vi "HFRR ADV v017 new software.vi"() -> ()   [LabVIEW 2025] (continued)
  # "µm"
  # "Calibration Centre\nSelect a calibration procedure to begin. Each procedure guides you through all required steps."
  # "Apply known deadweight loads to validate \nthe friction force measurement chain \nand compute the calibration factor for the f\norce transducer."
  # "Step-by-step guided displacement calibration \nacross 6 positions from 0.1 mm to 1.2 mm. Tear \nfirst, then measure each position one by one."
  # "Two-set calibration: one point at 0 °C \nice-point) and one at 60 °C (high-point) \nusing a  reference Calibrator."
  # "Step 1 — Pre-calibration Setup"
  # "Prepare the displacement calibration reference gauge. Ensure the LVDT sensor is connected and the carriage slides freely. You will be guided through 6 positions from 0.2 mm to 1.2 mm, one at a time"
  # "Step 7 — Tare ( ZERO REFERENCE )"
  # "Before measuring, the sensor must be zeroed. Move the carriage to the mechanical zero stop — no displacement applied. Once in position, tap Tare & Begin to zero the reference."
  # "Step 8 — POSITION MEASUREMENT"
  # "Measurement Checklist"
  # "Position the carriage at exactly this \nvalue using your reference gauge, then tap Confirm &\n Next."
  # "All 6 positions recorded!\n\nTap Confirm & Next  to review the calibration summary."
  # "Step 9 — CALIBRATION RESULT"
  # "Stroke Calibration Complete\nAll 6 positions (0.2 mm – 1.2 mm)"
  # "Calibrates the sample/bath temperature sensor. \nUsed for test specimen and lubricant temperature measurement."
  # "Calibrates the ambient air temperature sensor. \nUsed for environmental chamber monitoring."
  # "Set B\n60 °C\nHigh-point calibration"
  # "Set A\n0 °C\nIce-point calibration"
  # "Set B\n60 °C\nHigh-point calibration"
  # "Set A\n0 °C\nIce-point calibration"
  # "Select Temperature Sensor"
  # "Choose which temperature sensor you are calibrating. Both use the same two-\npoint procedure: 0 °C (ice-point) and 60 °C (high-point)."
  # "Step 1 — Reference Instrument Setup"
  # "Connect a calibrated reference to the DUT port. This calibration performs two sets: one at 0 °C and one at 60 °C."
  # "Set A\n0 °C\nIce-point calibration"
  # "Set B\n60 °C\nHigh-point calibration"
  # "Allow the temperature bath to stabilise for at least 2 minutes at each set-point before recording the reading."
  # "Step 2 — Set A:  0 °C Calibration"
  # "Connect the  0 °C reference connector. Wait for the temperature to stabilise. Once stable, and click Record Point."
  # "Step 3 — Set A:  60 °C Calibration"
  # "Connect the  60 °C reference connector. Wait for the temperature to stabilise. Once stable, and click Record Point."
  # "Step 1 — Reference Instrument Setup"
  # "Connect a calibrated reference to the DUT port. This calibration performs two sets: one at 0 °C and one at 60 °C."
  # "Set A\n0 °C\nIce-point calibration"
  # "Set B\n60 °C\nHigh-point calibration"
  # "Allow the temperature bath to stabilise for at least 2 minutes at each set-point before recording the reading."
  # "Step 2 — Set A:  0 °C Calibration"
  # "Connect the  0 °C reference connector. Wait for the temperature to stabilise. Once stable, and click Record Point."
  # "Step 3 — Set A:  60 °C Calibration"
  # "Connect the  60 °C reference connector. Wait for the temperature to stabilise. Once stable, and click Record Point."
  # "System Control Commands\nS;1 - Starts the full automation cycle (Runs Priming-humidify till 70RH sequence first, then switches to Maintenance).\nS;0 - Stops the system immediately and enters Standby mode (Safe State: All actuators OFF).\nM;1 - Skips the priming sequence and jumps directly to Maintenance mode (PID control).\nR;1 - Resets the logic state machine and clears all errors, returning to Standby.\nService Mode (Manual Control)\nX;1 - Enters Manual Service Mode. This disables all automatic logic, sensor safety checks, and timers.\nX;0 - Exits Manual Service Mode and returns to Standby (Safe State).\nActuator Commands (Only work after sending X;1)\nP;[0-255] - Sets the Pump PWM. Note that this is Active Low (0 = Max Flow, 255 = Pump OFF).\nF;I;[0-255] - Sets the Intake Fan speed (0 = OFF, 255 = Max Speed).\nF;O;[0-255] - Sets the Exhaust Fan speed (0 = OFF, 255 = Max Speed).\nD;1 - Turns the Dehumidifier Relay ON.\nD;0 - Turns the Dehumidifier Relay OFF."
  # "%RH"
  # "ISO : WS1.4"
  # "Start test and end test log--- done\nDisable heater ON and Humidity ON during the test --- done\ntemprature and ---done\nhumidity reach log\nauto start run true logic and log\nmanual start log once"
  # "Reference Fluid Information"
  # "Note:\nMake sure to place all images in the folder \"C:\\WinDucom\\im\" before clicking on \"Import Image.\""
  # "NOTE:\nPlace all the images in the path \"C:\\WinDucom\\im\" before clicking on Import Image"
  # "Wear Scar Measurements"
  # "Reference Fluid Information"
  # "Graph :"
types:
  T1 = enum32{"Home", "Dashboard", "Imaging", "Report", "Analysis", "About", "Test Setup", "Advance", "Calibration"}
  T2 = enum32{"HOME", "Test Setup", "Acquire", "Adv Scar", "Adv Scar Report", "Compare Files", "Calibration", "About", "Advance", "Mooha"}
  T3 = enum16{"ASTM D6079", "ISO 12156", "CEC F-096-A-06", "Custom"}
  T4 = enum32{"Dashboard 1", "Dashboard 2", "Dashboard 3"}
  T5 = enum32{"COF", "Friction", "ECR", "Temperature", "Humidity", "Stroke"}
  T6 = enum32{"Coefficient Of Friction", "Air Temperature", "Humidity", "Stroke", "Sample Temperature", "Electrical Contact Resistance", "Frequency", "Air Temp vs Rh"}
  T7 = enum32{"Main", "Stroke", "Friction", "Temperature"}
  T8 = enum32{"Stroke Calibration", "Friction Force Calibration", "Temperature Calibration"}
  T9 = enum32{"Step 1", "Step 2", "Step 3", "Step 4", "Step 5", "Step 6", "Step 7", "Step 8", "Step 9"}
  T10 = enum32{"Test Progress", "Stroke Points Completed"}
  T11 = enum32{"Main", "Step 1", "Step 2", "Step 3", "Air Step 1", "Air Step 2", "Air Step 3"}
  T12 = enum32{"Gains", "Configuration Parameters", "Temperature Calibration"}
  T13 = enum32{"Stroke Data", "Temperature Calibration", "Friction Force Raw Data"}
  T14 = enum32{"Temp Variables", "Camera", "WO 2465 (1)", "WO 2465 (2)", "WO 2465 (3)"}
  T15 = typedef "Auto Start enum.ctl" = enum16{"Init", "Humidity & Temperature On", "Reach point", "Maintain Stage", "Start Stage", "close", "Exit"}
  T16 = typedef "imagedata.ctl" = cluster{"image type":i32, "image depth":i32, "image":u8[], "mask":u8[], "colors":u32[], "Rectangle":cluster{"left":i16, "top":i16, "right":i16, "bottom":i16}}
  T17 = enum32{"HOME", "Test Setup", "Acquire", "Compare Files", "Print Report", "About", "Advance", "Mooha"}
  T18 = cluster{"Read Heave and Surge":string, "Bytes at Heave Port":dbl, "Heave and Surge COM Port:":refnum<visa-resource-name>, "Com Port 2":refnum<visa-resource-name>, "Residual Due":string, "Heave COM Status 2":bool, "Heave COM Status":bool, "Port 2":bool, "Sway PPR":dbl, "Surge PPR":dbl, "Heave PPR":dbl, "Sway Pitch":dbl, "Surge Pitch":dbl, "Heave Pitch":dbl, "Sway Pulses/mm":dbl, "Surge Pulses/mm":dbl, "Heave Pulses/mm":dbl, "inner loop":dbl, "Read Heave and Surge 2":string, "String 36":string, "Write S":bool, "WriteCC1":string[], "Heave COM Loop":i32, "LastCom":string, "EXIT":bool, "Error Heave":errorcluster}
  T19 = enum8{"Enabled", "Disabled", "Disabled and Grayed Out"}
  T20 = enum32{"HOME", "Test Setup", "Acquire", "Adv Scar", "Adv Scar Report", "Compare Files", "About", "Advance", "Mooha"}
  T21 = enum16{"Always On", "Always Off", "Off While Running"}
  T22 = typedef "POST ANALYSIS ENUM.ctl" = enum16{"OPEN EXE", "INIT", "OPEN FILE", "FIT", "DRAW REC", "DRAW LINE", "PAN", "ZOOM IN", "ZOOM OUT", "SET ZOOM", "CLEAR ROI", "GET MEASUREMENTS", "RESIZE MODE", "STREAM START", "STREAM STOP", "SHOW UI", "MINIMIZE UI", "HIDE UI", "CKISE APP", "CLOSE CONNECTION", "SAVE IMAGE", "SET ROI COLOR", "READ", "TCP CHECK", "CLOSE"}
  T23 = typedef "CAMERA LIVE FEED ENUM.ctl" = enum16{"OPEN EXE", "INIT", "READ", "CAMERA CONNECT", "CAMERA START", "CAMERA STOP", "CAMERA GRAY", "CAMERA RGB", "CAMERA MINIMIZE", "CAMERA CLOSE", "CAMERA MODE LIST", "CAMERA MODE SET", "CAMERA RESTORE", "CAMERA SAVE", "CLOSE"}
  T24 = enum32{"Home", "Dashboard", "Imaging", "Report", "Analysis", "About", "Test Setup", "Advance"}
  T25 = cluster{"File Name":string, "Test Method":string, "Operator":string, "Fuel Description":string, "Date and time":string}
  T26 = enum32{"Home", "Dashboard", "Imaging", "Report", "Analysis", "About", "Test Setup"}
  T27 = enum32{"HOME", "Test Setup", "Acquire", "Compare Files", "About", "Advance", "Mooha"}
  T28 = enum16{"deny read/write", "deny write-only", "deny none"}
  T29 = typedef "NI_ReportGenerationCore.lvlib/HTML Report Image Alignment.ctl" = enum16{"(default)", "LEFT", "RIGHT", "TOP", "TEXTTOP", "MIDDLE", "ABSMIDDLE", "BASELINE", "BOTTOM", "ABSBOTTOM"}
  T30 = enum16{"open", "replace", "create", "open or create", "replace or create", "replace or create with confirmation"}
  T31 = enum16{"INIT", "READ", "MANUAL WRITE", "WRITE", "CLOSE", "ERROR INIT"}
  T32 = enum16{"open", "open or create", "create or replace", "create", "open (read only)"}
  T33 = cluster{"Mode":enum16{"RTU", "ASCII"}, "Slave Address":u8}
diagram:
  w11 = FALSE ("Visible")
  w12 = T19."Enabled" ("Disabled")
  w15 = FALSE ("Visible")
  w14 = FALSE ("Humidity Off Command")
  w32 = "" ("USER ID")
  (unwired) T20."HOME" ("Main Tab")
  # "[CH1]    - FF\n[CH2]   - TEMPERATURE\n[CH3]    - Humidity\n[CH4]    - AIR TEMP\n[CH5]\\- Visa Uno\n[CH6] \\- Visa Due\n[CH7]  \\- file path\n[CH8]   - Displacement Gain\n[CHA]   - Stroke Gain\n[CHB]   - Stroke PID Gain\n[CHC]   -Language Selection\n[CHD]   -Power +\n[CHE]   -Power_\n[CHF]   -Heater\n[CHG]   -Humidity Wet\n[CHH]   -Humidity Dry\n[CHI]   -Integral Time \n[CHIJ   -Air intercept\n[CHI]   -Temp Intercept"
  n1 = flat-sequence {
    tunnel: [w81] -> w24
    tunnel: w24 -> [w95]
    tunnel: [w94] -> w23
    tunnel: ["ao0"] -> w26
    tunnel: w23 -> [_]
    tunnel: w26 -> [w159]
    tunnel: [w159] -> w25
    tunnel: w25 -> [w205]
    tunnel: [w203] -> w36
    tunnel: [w205] -> w35
    tunnel: w36 -> [w255]
    tunnel: w35 -> [w212]
    tunnel: [w255] -> w22
    tunnel: [w218] -> w21
    tunnel: [w206] -> w20
    tunnel: [w261] -> _
    tunnel: [w260] -> _
    tunnel: [w262] -> w58
    tunnel: w22 -> [w262]
    tunnel: w21 -> [w260]
    tunnel: w20 -> [w261]
    frame #0 {
      n2 = disable-structure shown="Disabled" {
        frame Disabled {
          n3 = control-ref of="This VI"() -> (w69:refnum<vi>)
          n4 = property class="VI"(reference=w69) -> (reference out=w60:refnum<vi>, error out=w64:errorcluster, "Panel"=w68:refnum<vi>)  [unwired: 1 in]
          n5 = property class="Pnl"(reference=w68, error in=w64) -> (reference out=w62:refnum<vi>, error out=w65:errorcluster, "Panes[]"=w67:refnum<vi>[])
          n6 = for {
            tunnel: w67 -> [w75] mode=indexing
            tunnel: T21."Always Off" ("Horizontal Scrollbar Visibility") -> [w74]
            tunnel: w65 -> [w71]
            tunnel: [w70] -> w63
            n7 = property class="Pane"(reference=w75, error in=w71, "HorizScrollbarVisibility"=w74) -> (reference out=w72:refnum<vi>, error out=w73:errorcluster)
            n8 = Close Reference(reference=w72, error in (no error)=w73) -> (error out=w70:errorcluster)
          }
          n9 = Close Reference(reference=w62, error in (no error)=w63) -> (error out=w61:errorcluster)
          n10 = Close Reference(reference=w60, error in (no error)=w61) -> (error out=→"error out 8":errorcluster)
        }
        frame Enabled {
        }
      }
    }
    frame #1 {
      n11 = call "CLOSE CONNECTION.vi"("error in (no error)"="error in (no error) 2") -> ("error out"=w79:errorcluster)  [unwired: 10 in]
      n12 = call <vilib>:"Clear Errors.vi"("error in (no error)"=w79) -> ("error out"=w78:errorcluster)  [unwired: 5 in, 1 out]
      n13 = disable-structure shown="Enabled" {
        disable-tunnel: w78 -> [w85 _]
        disable-tunnel: [w84 _] -> w81
        frame Enabled {
          n14 = call <userlib>:"Fit VI window to Largest Dec.vi"("error in (no error)"=w85, "border spacing (2 px)"=1) -> ("error out"=w88:errorcluster, "dup VI Ref"=w92:refnum<vi>)  [unwired: 4 in]
          n15 = invoke on="Invoke Node" class="VI" method="FP.Run-Time Position.Maximized"(reference=w92, error in=w88) -> (error out=w89:errorcluster)  [unwired: 2 in, 3 out]
          n16 = call <vilib>:"Clear Errors.vi"("error in (no error)"=w89) -> ("error out"=w91:errorcluster)  [unwired: 5 in, 1 out]
          n17 = control-ref of="This VI"() -> (w83:refnum<vi>)
          n18 = invoke on="Invoke Node" class="VI" method="Default Vals.Reinit All"(reference=w83, error in=w91) -> (reference out=w87:refnum<vi>, error out=w86:errorcluster)  [unwired: 1 in, 1 out]
          n19 = Close Reference(reference=w87, error in (no error)=w86) -> (error out=w84:errorcluster)
        }
        frame Disabled {
        }
      }
      n20 = local write "sign in temp"(FALSE ("sign in temp")) -> ()
      n21 = property on="Sign In" class="Bool (strict)"("DisabledEnum"=T19."Disabled" ("Disabled")) -> ()  [unwired: 2 in, 2 out]
      n22 = property on="Auto Scar Check" class="Clust (strict)"("Visible"=TRUE) -> ()  [unwired: 2 in, 2 out]
    }
    frame #2 {
      n23 = call "dialog box.vi"("Status"="Before starting the test, verify that the microscope cable is connected.", "error in"=w95) -> ("error out"=w94:errorcluster)  [unwired: 8 in]
    }
    frame #3 {
      (unwired) TRUE ("Re-Initialise")
      w101 = FALSE ("Upld AR 2")
      # "kkkkk"
      # "C:\\Windows\\wndcm_pw_stdED hfrr.txt"
      # "C:\\LAB-IQ NXT"
      # "C:\\LAB-IQ NXT\\wndcm_pw_stdED hfrr.txt"
      # "password file"
      n24 = Current VI's Path() -> (path=w114:path)
      n25 = Strip Path(path=w114) -> (stripped path=w107:path)  [unwired: 1 out]
      n26 = Path To String(path=w107) -> (string=w109:string)
      n27 = local write "conststatus"(0.0 ("rpm value : 2")) -> ()
      n28 = local write "Upld AR 2"(TRUE ("Upld AR 2")) -> ()
      n29 = local write "Lan flag"(0.0 ("Lan flag")) -> ()
      n30 = local write "COUNT"(0 ("COUNT")) -> ()
      n31 = local write "FLAG 2"(0.0 ("FLAG 2")) -> ()
      n32 = local write "Com flag"(u32 0 ("Com flag")) -> ()
      n33 = local write "refresh flag"(FALSE ("refresh flag")) -> ()
      n34 = local write "Json St Flg"(w101) -> ()
      n35 = Search/Split String(string=w109, search string/char (-)=".exe") -> (match + rest of string=w111:string)  [unwired: 1 in, 2 out]
      n36 = Match True/False String(2:".vi" ("false string"), 3:".exe" ("true string"), 4:w111) -> (0:w108:bool)  [unwired: 1 out]
      n37 = local write "Json End Flg"(w101) -> ()
      n38 = case shown="True" w108 {
        tunnel: w107 -> [w130 w132]
        tunnel: [w130 w131] -> w105
        frame False {
        }
        frame True {
          n39 = Strip Path(path=w132) -> (stripped path=w131:path)  [unwired: 1 out]
        }
      }
      n40 = Path To String(path=w105) -> (string=→"Gain path":string)
      n41 = local write "Main Tab Display"(T4."Dashboard 1" ("Main Tab Display")) -> ()
      n42 = local write "main tab sub"(enum32{"Page 1", "Page 2"}."Page 1" ("main tab sub")) -> ()
      n43 = local write "Main Tab"(T2."HOME" ("Main Tab")) -> ()
      n44 = local write "EVENT LOG"("") -> ()
      n45 = List Folder(path=path "C:/LAB-IQ" ("directory path"), pattern="*.txt") -> (filenames=w120:string[])  [unwired: 2 in, 3 out]
      n46 = Search 1D Array(1D array=w120, element="wndcm_pw_stdED hfrr.txt") -> (index of element=w123:i32)  [unwired: 1 in]
      n47 = Equal?(x=w123, y=-1) -> (x = y?=w118:bool)
      n48 = case shown="True" w118 {
        frame False {
        }
        frame True {
          n49 = String To Byte Array(string="123\n") -> (unsigned byte array=w137:u8[])
          n50 = Array Size(array=w137) -> (size(s)=w136:i32)
          n51 = for {
            N: w136 -> [_]
            tunnel: w137 -> [w150]
            tunnel: [w147] -> w139 mode=indexing
            tunnel: w136 -> [w142]
            i -> [w140]
            n52 = Decrement(x=w142) -> (x-1=w143:i32)
            n53 = Equal?(x=w140, y=w143) -> (x = y?=w144:bool)
            n54 = Index Array(array=w150, index=w140) -> (element=w149:u8)
            n55 = Number To Decimal String(number=w149) -> (decimal integer string=w148:string)  [unwired: 1 in]
            n56 = Select(t="", s=w144, f="\r") -> (s? t:f=w141:string)
            n57 = Concatenate Strings(w148, w141) -> (w147:string)
          }
          n58 = local read "file path"() -> (w133:path)
          n59 = Concatenate Strings(w139) -> (w135:string)
          n60 = call <vilib>:"Write Characters To File.vi"("append to file? (new file:F)"=FALSE, "character string"=w135, "file path (dialog if empty)"=w133) -> ()  [unwired: 2 in, 1 out]
        }
      }
      n61 = local write "clk"(0.0 ("clk")) -> ()
      n62 = local write "Flag"(0.0 ("Flag")) -> ()
      "file path" <- path "C:/LAB-IQ/wndcm_pw_stdED hfrr.txt" ("file path")
      "FF buffer" <- dbl[] [] ("FF buffer")
    }
    frame #4 {
      # "C:\\WinDucom\\calibrate WO 2391.dcf"
      n63 = String To Path(string="C:\\LAB-IQ\\calibrate WO 2465.dcf") -> (path=w158:path)
      n64 = Open/Create/Replace File "Open File"(file path (use dialog)=w158) -> (refnum out=w157:refnum<file>)  [unwired: 5 in, 2 out]
      n65 = for {
        N: 24 -> [_]
        tunnel: w157 -> [w178]
        i -> [w172]
        (unwired) TRUE ("line mode (F)")
        n66 = Read from Text File "Read File"(file (use dialog)=w178) -> (text=w177:string)  [unwired: 3 in, 3 out]
        n67 = Match Pattern(string=w177, regular expression="]") -> (after substring=w175:string)  [unwired: 1 in, 3 out]
        n68 = String Subset(string=w177, offset (0)=5, length (rest)=10 ("length (rest)")) -> (substring=w170:string)
        n69 = Fract/Exp String To Number(string=w170) -> (number=w171:dbl)  [unwired: 3 in, 1 out]
        n70 = Match Pattern(string=w175, regular expression="-") -> (before substring=w173:string)  [unwired: 1 in, 3 out]
        n71 = case shown="19" w172 {
          tunnel: w171 -> [w181 w182 w183 w184 _ _ _ w189 w190 _ w191 w192 w193 w194 w195 w196 _ w197 w198 _ _ _ _ _ _]
          tunnel: w173 -> [_ _ _ _ w185 w186 w187 _ _ _ _ _ _ _ _ _ _ _ _ w199 w200 _ w201 w202 _]
          frame 0 {
            n72 = local write "FRIC. FORCE :"(w181) -> ()
          }
          frame 1 {
            n73 = local write "TEMPERATURE :"(w182) -> ()
          }
          frame 2 {
            n74 = local write "HUMIDITY:"(w183) -> ()
          }
          frame 3 {
            n75 = local write "AIR TEMPERATURE :"(w184) -> ()
          }
          frame 4 {
            n76 = local write "Com Port 1"(w185) -> ()
          }
          frame 5 {
            n77 = local write "Com Port 2"(w186) -> ()
            n78 = local write "visa due"(w186) -> ()
          }
          frame 6 {
            n79 = String To Path(string=w187) -> (path=w188:path)
            n80 = local write "File Path"(w188) -> ()
          }
          frame 7 {
            n81 = local write "DISPLACEMENT :"(w189) -> ()
          }
          frame 8 {
            n82 = local write "STROKE GAIN :"(w190) -> ()
          }
          frame 9 {
          }
          frame 10 {
            n83 = local write "Language Selection"(w191) -> ()
          }
          frame 11 {
            n84 = local write "CH-POWER +"(w192) -> ()
          }
          frame 12 {
            n85 = local write "CH-POWER -"(w193) -> ()
          }
          frame 13 {
            n86 = local write "CH-HEATER"(w194) -> ()
          }
          frame 14 {
            n87 = local write "CH-HUMIDITY WET"(w195) -> ()
          }
          frame 15 {
            n88 = local write "CH-HUMIDITY DRY"(w196) -> ()
          }
          frame 16 {
          }
          frame 17 {
            n89 = local write "AIR TEMP INTERCEPT:"(w197) -> ()
          }
          frame 18 {
            n90 = local write "TEMP INTERCEPT:"(w198) -> ()
          }
          frame 21 {
            n91 = local write "S.NO"(w199) -> ()
          }
          frame 22 {
            n92 = local write "Com Port 3"(w200) -> ()
          }
          frame 23 {
          }
          frame 19 {
            n93 = local write "C3 :"(w201) -> ()
          }
          frame 20 {
            n94 = local write "Camera Port :"(w202) -> ()
          }
          frame 24, Default {
          }
        }
      }
      n95 = String To Path(string="C:\\LAB-IQ\\Image Calibrate v01.dcf") -> (path=w154:path)
      n96 = Open/Create/Replace File ("Open File")(file path (use dialog)=w154) -> (refnum out=w153:refnum<file>)  [unwired: 5 in, 2 out]
      n97 = for {
        N: 4 -> [_]
        tunnel: w153 -> [w165]
        i -> [w161]
        n98 = Read from Text File ("Read File")(file (use dialog)=w165) -> (text=w166:string)  [unwired: 3 in, 3 out]
        n99 = String Subset(string=w166, offset (0)=6, length (rest)=10 ("length (rest)")) -> (substring=w162:string)
        n100 = Fract/Exp String To Number(string=w162) -> (number=w160:dbl)  [unwired: 3 in, 1 out]
        n101 = case shown="3" w161 {
          tunnel: w160 -> [w167 w168 _ w169 _]
          frame 0 {
            n102 = local write "5x Gain"(w167) -> ()
          }
          frame 1 {
            n103 = local write "10x Gain"(w168) -> ()
          }
          frame 2 {
          }
          frame 3 {
            n104 = local write "100x gain"(w169) -> ()
          }
          frame 4, Default {
          }
        }
      }
    }
    frame #5 {
      n105 = Wait (ms)(milliseconds to wait=u32 1000) -> (millisecond timer value=w203:u32)
    }
    frame #6 {
      w221 = u32 2000 ("milliseconds to wait")
      w248 = u32 2000 ("milliseconds to wait")
      n106 = call "CAMERA LIVE FEED FGV.vi"("Enum - Menu"=CAMERA_LIVE_FEED_ENUM."OPEN EXE", "error in (no error)"=w212) -> ("error out"=w254:errorcluster)  [unwired: 8 in, 1 out]
      n107 = call "Stall Data Flow.vim"("value in"=w254, "milliseconds to wait"=w248) -> ("value out"=w252:errorcluster)  [unwired: 1 out]
      n108 = call "CAMERA LIVE FEED FGV.vi"("Enum - Menu"=CAMERA_LIVE_FEED_ENUM."INIT", "error in (no error)"=w252) -> ("error out"=w250:errorcluster)  [unwired: 8 in, 1 out]
      n109 = call "IMAGE ANALYSIS.vi"("Enum"=POST_ANALYSIS_ENUM."OPEN EXE", "error in"=w212) -> ("error out"=w209:errorcluster)  [unwired: 8 in, 1 out]
      n110 = case shown="Error .." w250 {
        selector: w250 -> [w256 _]
        tunnel: [w256 _] -> w249
        frame No Error {
        }
        frame Error {
          n111 = One Button Dialog(message="Camera initialization error.\nPlease Restart the software") -> ()  [unwired: 1 in, 1 out]
        }
      }
      n112 = call "Stall Data Flow.vim"("value in"=w209, "milliseconds to wait"=u32 8000) -> ("value out"=w208:errorcluster)  [unwired: 1 out]
      n113 = property on="Camera Port :" class="CmbBox"() -> ("Strings[]"=w246:string[], "Value"=w247:string)  [unwired: 2 in, 2 out]
      n114 = call "IMAGE ANALYSIS.vi"("Enum"=POST_ANALYSIS_ENUM."INIT", "error in"=w208) -> ("error out"=w206:errorcluster)  [unwired: 8 in, 1 out]
      n115 = Search 1D Array(1D array=w246, element=w247) -> (index of element=w245:i32)  [unwired: 1 in]
      n116 = Type Cast(type=30, x=w245) -> (*(type *) &x=w243:i32)
      n117 = call "Stall Data Flow.vim"("value in"=w249, "milliseconds to wait"=w248) -> ("value out"=w225:errorcluster)  [unwired: 1 out]
      n118 = Add(x=w243, y=48) -> (x+y=w224:i32)
      n119 = call "CAMERA LIVE FEED FGV.vi"("Enum - Menu"=CAMERA_LIVE_FEED_ENUM."CAMERA CONNECT", "error in (no error)"=w225, "CAMERA PORT"=w224) -> ("error out"=w234:errorcluster)  [unwired: 7 in, 1 out]
      n120 = call "Stall Data Flow.vim"("value in"=w234, "milliseconds to wait"=u32 5000) -> ("value out"=w235:errorcluster)  [unwired: 1 out]
      n121 = call "CAMERA LIVE FEED FGV.vi"("Enum - Menu"=CAMERA_LIVE_FEED_ENUM."CAMERA MODE LIST", "error in (no error)"=w235) -> ("error out"=w237:errorcluster)  [unwired: 8 in, 1 out]
      n122 = call "Stall Data Flow.vim"("value in"=w237, "milliseconds to wait"=w221) -> ("value out"=w236:errorcluster)  [unwired: 1 out]
      n123 = call "CAMERA LIVE FEED FGV.vi"("Enum - Menu"=CAMERA_LIVE_FEED_ENUM."READ", "error in (no error)"=w236) -> ("error out"=w223:errorcluster, "data out"=→"Camera List":string)  [unwired: 8 in]
      n124 = call "Stall Data Flow.vim"("value in"=w223, "milliseconds to wait"=w221) -> ("value out"=w222:errorcluster)  [unwired: 1 out]
      n125 = Type Cast(type=30, x=0) -> (*(type *) &x=w217:i32)
      n126 = Add(x=w217, y=48) -> (x+y=w215:i32)
      n127 = call "CAMERA LIVE FEED FGV.vi"("Enum - Menu"=CAMERA_LIVE_FEED_ENUM."CAMERA MODE SET", "error in (no error)"=w222, "CAMERA MODE"=w215) -> ("error out"=w219:errorcluster)  [unwired: 7 in, 1 out]
      n128 = call "Stall Data Flow.vim"("value in"=w219, "milliseconds to wait"=u32 2000) -> ("value out"=w239:errorcluster)  [unwired: 1 out]
      n129 = call "CAMERA LIVE FEED FGV.vi"("Enum - Menu"=CAMERA_LIVE_FEED_ENUM."CAMERA START", "error in (no error)"=w239) -> ("error out"=w240:errorcluster)  [unwired: 8 in, 1 out]
      n130 = call "Stall Data Flow.vim"("value in"=w240, "milliseconds to wait"=u32 1000) -> ("value out"=w241:errorcluster)  [unwired: 1 out]
      n131 = call "CAMERA LIVE FEED FGV.vi"("Enum - Menu"=CAMERA_LIVE_FEED_ENUM."CAMERA MINIMIZE", "error in (no error)"=w241) -> ("error out"=w218:errorcluster)  [unwired: 8 in, 1 out]
    }
    frame #7 {
      n132 = case shown="No Error" w260 {
        frame No Error {
          n133 = property on="Auto Scar Check" class="Clust (strict)"("Visible"=FALSE) -> ()  [unwired: 2 in, 2 out]
        }
        frame Error {
        }
      }
      n134 = local write "sign in temp"(TRUE ("sign in temp")) -> ()
      n135 = property on="Sign In" class="Bool (strict)"("DisabledEnum"=T19."Enabled" ("Disabled")) -> ()  [unwired: 2 in, 2 out]
    }
  }
  n136 = local write "Cal Password"("" ("Cal Password")) -> ()
  n137 = property on="Auto Start Test" class="Bool (strict)"("Visible"=TRUE) -> ()  [unwired: 2 in, 2 out]
  n138 = property on="FRICVALZ 2" class="Bool (strict)"("DisabledEnum"=w12) -> ()  [unwired: 2 in, 2 out]
  n139 = property on="FRICVALZ 4" class="Bool (strict)"("DisabledEnum"=w12) -> ()  [unwired: 2 in, 2 out]
  n140 = property on="FRICVALZ 3" class="Bool (strict)"("DisabledEnum"=w12) -> ()  [unwired: 2 in, 2 out]
  n141 = property on="About" class="Clust (strict)"("Visible"=FALSE) -> ()  [unwired: 2 in, 2 out]
  n142 = property on="Tab Control 5" class="TabCtl (strict)"("Tabs Visible?"=TRUE ("Page Labels Display Visible?")) -> ()  [unwired: 2 in, 2 out]
  n143 = property on="Wrong Password" class="Str"("Visible"=w11) -> ()  [unwired: 2 in, 2 out]
  n144 = property on="Calibration 2" class="TabCtl (strict)"("Visible"=w11) -> ()  [unwired: 2 in, 2 out]
  n145 = local write "SCAR MEASURMENT"(enum32{"Auto Scar", "Manual Scar"}."Manual Scar" ("SCAR MEASURMENT")) -> ()
  n146 = local write "Temperature Off Command"(w14) -> ()
  n147 = local write "Main Dashboard Buttons"(T1."Home" ("Main Dashboard Buttons")) -> ()
  n148 = local write "Humidity Off Command"(w14) -> ()
  n149 = local write "CAMERA ROI MIN TEMP"(w14) -> ()
  n150 = local write "TEST FILE NAM,E SAVED"(w14) -> ()
  n151 = local write "LIVE FEED MIN TEMP"(w14) -> ()
  n152 = local write "SCAR MEASURMENT"(enum32{"Auto Scar", "Manual Scar"}."Manual Scar" ("SCAR MEASURMENT")) -> ()
  n153 = local write "Auto stop temp"(w15) -> ()
  n154 = local write "main tab sub"(enum32{"Page 1", "Page 2"}."Page 1" ("main tab sub")) -> ()
  n155 = local write "USERNAME"(w32) -> ()
  n156 = local write "Main Tab"(T2."HOME" ("Main Tab")) -> ()
  n157 = local write "USER ID"(w32) -> ()
  n158 = property on="Auto Scar Check  2" class="Clust (strict)"("Visible"=w15) -> (error out=w18:errorcluster)  [unwired: 2 in, 1 out]
  n159 = property on="Quit" class="Bool (strict)"("Value"=FALSE ("Quit")) -> (error out=w34:errorcluster)  [unwired: 2 in, 1 out]
  n160 = while {
    stop <- w264 stop-if-true
    n161 = event shown="[36] \"Temperature Continue Step 3\": Value Change" {
      selector: _ -> [_ _ _ _ _ _ _ _ _ _ _ _ _ _ _ _ _ _ _ _ _ _ _ _ _ _ _ _ _ _ _ _ _ _ _ _ _ _ _]
      dyn-events: _ -> [_ _ _ _ _ _ _ _ _ _ _ _ _ _ _ _ _ _ _ _ _ _ _ _ _ _ _ _ _ _ _ _ _ _ _ _ _ _ _]
      timeout: 100 -> [_ _ _ _ _ _ _ _ _ _ _ _ _ _ _ _ _ _ _ _ _ _ _ _ _ _ _ _ _ _ _ _ _ _ _ _ _ _ _]
      tunnel: [FALSE FALSE _ FALSE _ _ _ _ _ _ _ _ _ _ _ _ _ _ _ _ _ _ _ _ _ _ _ _ _ _ _ _ _ _ _ _ _ _ TRUE] -> w264
      event Timeout {
        n162 = event-data() -> ()  [unwired: 1 in, 3 out]
        n163 = disable-structure shown="Disabled" {
          frame Disabled {
            n164 = local read "Auto Start Test"() -> (w278:bool)
            n165 = local read "RUN"() -> (w279:bool)
            n166 = Or(x=w279, y=w278) -> (x .or. y?=w277:bool)
            n167 = case shown="True" w277 {
              frame False {
                w280 = TRUE ("PAUSE")
                n168 = call "ELAPSED TIMER VI - abort test.vi"("RESET"=w280, "PAUSE"=w280) -> ()  [unwired: 7 in, 3 out]
              }
              frame True {
                n169 = local read "Stroke 2"() -> (w285:dbl)
                n170 = local read "FF 3"() -> (w287:dbl)
                n171 = Equal?(x=w285, y=0.95 ("Stroke 2")) -> (x = y?=w282:bool)
                n172 = Equal?(x=w287, y=0.0 ("FF 3")) -> (x = y?=w283:bool)
                n173 = Or(x=w283, y=w282) -> (x .or. y?=w281:bool)
                n174 = case shown="True" w281 {
                  selector: w281 -> [_ w292]
                  frame False {
                    w288 = TRUE ("PAUSE")
                    n175 = call "ELAPSED TIMER VI - abort test.vi"("RESET"=w288, "PAUSE"=w288) -> ()  [unwired: 7 in, 3 out]
                  }
                  frame True {
                    n176 = Not(x=w292) -> (.not. x?=w291:bool)
                    n177 = call "ELAPSED TIMER VI - abort test.vi"("TARGET"=60.0, "RESET"=w291, "PAUSE"=FALSE) -> ("ELAPSED INDICATION"=w289:bool)  [unwired: 6 in, 2 out]
                    n178 = case shown="True" w289 {
                      frame False {
                      }
                      frame True {
                        n179 = stacked-sequence {
                          frame #0 {
                            w294 = FALSE
                            n180 = local write "RUN"(w294) -> ()
                            n181 = local write "Auto Start Test"(w294) -> ()
                          }
                          frame #1 {
                            n182 = One Button Dialog(message="Test stopped due to a communication error. Reconnect the C1 and C2 cables.") -> ()  [unwired: 1 in, 1 out]
                          }
                        }
                      }
                    }
                  }
                }
              }
            }
          }
          frame Enabled {
          }
        }
        n183 = Get Date/Time In Seconds() -> (seconds since 1Jan1904=w275:timestamp)
        n184 = Format Into String(format string="%<%I:%M:%S:%p %d:%B:%Y>T", w275) -> (resulting string=→"Time Stamp":string)  [unwired: 2 in, 1 out]
        n185 = local read "Service Password enable"() -> (w267:bool)
        n186 = local read "FILE"() -> (w272:string)
        n187 = call <vilib>:"Trim Whitespace.vi"("string"=w272) -> ("trimmed string"=w271:string)  [unwired: 1 in]
        n188 = String Length(string=w271) -> (length=w270:i32)
        n189 = Greater?(x=w270, y=1) -> (0:w268:bool)
        n190 = case shown="False" w268 {
          tunnel: w267 -> [w296 _]
          frame False {
            n191 = case shown="False" w296 {
              frame True {
                w297 = "Test Start In Service Mode" ("Tip Strip")
                w298 = T19."Enabled" ("Disabled")
                n192 = property on="Auto Start Test" class="Bool (strict)"("DisabledEnum"=w298, "TipStrip"=w297) -> ()  [unwired: 2 in, 2 out]
                n193 = property on="RUN" class="Bool (strict)"("DisabledEnum"=w298, "TipStrip"=w297) -> ()  [unwired: 2 in, 2 out]
              }
              frame False {
                w299 = "Enter File Name to Start Test" ("Tip Strip")
                w300 = T19."Disabled and Grayed Out" ("Disabled")
                n194 = property on="Auto Start Test" class="Bool (strict)"("DisabledEnum"=w300, "TipStrip"=w299) -> ()  [unwired: 2 in, 2 out]
                n195 = property on="RUN" class="Bool (strict)"("DisabledEnum"=w300, "TipStrip"=w299) -> ()  [unwired: 2 in, 2 out]
              }
            }
          }
          frame True {
            w301 = "" ("Tip Strip")
            w302 = T19."Enabled" ("Disabled")
            n196 = property on="Auto Start Test" class="Bool (strict)"("DisabledEnum"=w302, "TipStrip"=w301) -> ()  [unwired: 2 in, 2 out]
            n197 = property on="RUN" class="Bool (strict)"("DisabledEnum"=w302, "TipStrip"=w301) -> ()  [unwired: 2 in, 2 out]
          }
        }
      }
      event "RUN": Value Change {
        n198 = event-data() -> ()  [unwired: 1 in, 6 out]
        n199 = local read "RUN"() -> (w304:bool)
        n200 = case shown="False" w304 {
          frame False {
            n201 = flat-sequence {
              frame #0 {
                n202 = local write "START TEMP"(FALSE ("START TEMP")) -> ()
              }
              frame #1 {
                n203 = Wait (ms)(milliseconds to wait=u32 1500) -> ()  [unwired: 1 out]
              }
              frame #2 {
              }
              frame #3 {
                n204 = local write "Command"("VC;0") -> ()
              }
              frame #4 {
                n205 = Wait (ms)(milliseconds to wait=u32 1500) -> ()  [unwired: 1 out]
              }
              frame #5 {
                w313 = T19."Enabled" ("Disabled")
                (unwired) T24."Imaging" ("Main Dashboard Buttons")
                (unwired) T20."Adv Scar" ("Main Tab")
                w315 = "" ("FILE")
                n206 = local write "measured_stroke"(0.0 ("measured_stroke")) -> ()
                n207 = local write "Command"("VC;0") -> ()
                n208 = local write "FILE"(w315) -> ()
                n209 = local write "Batch Ref Num :"(w315) -> ()
                n210 = local write "Fuel Discription :"(w315) -> ()
                n211 = local write "Main Tab"(T2."Adv Scar" ("Main Tab")) -> ()
                n212 = local write "Remarks :"(w315) -> ()
                n213 = local write "Main Dashboard Buttons"(T1."Imaging" ("Main Dashboard Buttons")) -> ()
                n214 = local write "TEST FILE NAM,E SAVED"(FALSE ("TEST FILE NAM,E SAVED")) -> ()
                n215 = property on="Stroke ( mm )" class="WFChart (strict)"("History Data"=cluster{"y":dbl, dbl, "y":dbl}[] []) -> ()  [unwired: 2 in, 2 out]
                n216 = property on="Auto Start Test" class="Bool (strict)"("Visible"=TRUE) -> ()  [unwired: 2 in, 2 out]
                n217 = property on="FRICVALZ 2" class="Bool (strict)"("DisabledEnum"=w313) -> ()  [unwired: 2 in, 2 out]
                n218 = property on="FRICVALZ 4" class="Bool (strict)"("DisabledEnum"=w313) -> ()  [unwired: 2 in, 2 out]
                n219 = property on="FRICVALZ 3" class="Bool (strict)"("DisabledEnum"=w313) -> ()  [unwired: 2 in, 2 out]
              }
            }
          }
          frame True {
            n220 = flat-sequence {
              frame #0 {
                n221 = local write "Command"("VC;1") -> ()
              }
              frame #1 {
                n222 = Wait (ms)(milliseconds to wait=u32 2000) -> ()  [unwired: 1 out]
              }
              frame #2 {
                n223 = local write "Command"("VC;1") -> ()
              }
              frame #3 {
                n224 = Wait (ms)(milliseconds to wait=u32 2000) -> ()  [unwired: 1 out]
              }
              frame #4 {
                w323 = T19."Disabled" ("Disabled")
                n225 = property on="Auto Start Test" class="Bool (strict)"("Visible"=FALSE) -> ()  [unwired: 2 in, 2 out]
                n226 = local write "START TEMP"(TRUE ("START TEMP")) -> ()
                n227 = property on="FRICVALZ 2" class="Bool (strict)"("DisabledEnum"=w323) -> ()  [unwired: 2 in, 2 out]
                n228 = property on="FRICVALZ 4" class="Bool (strict)"("DisabledEnum"=w323) -> ()  [unwired: 2 in, 2 out]
                n229 = property on="FRICVALZ 3" class="Bool (strict)"("DisabledEnum"=w323) -> ()  [unwired: 2 in, 2 out]
              }
            }
          }
        }
      }
      event "Auto": Value Change {
        n230 = event-data() -> ()  [unwired: 1 in, 6 out]
        n231 = stacked-sequence {
          frame #0 {
            n232 = local write "FILE"("") -> ()
          }
          frame #1 {
            n233 = Get Date/Time In Seconds() -> (seconds since 1Jan1904=w329:timestamp)
            n234 = Format Into String(format string="%<%I_%M_%S_%p_%d_%B_%Y>T", w329) -> (resulting string=w328:string)  [unwired: 2 in, 1 out]
            n235 = local write "FILE"(w328) -> ()
          }
        }
        n236 = local read "Auto"() -> (w326:bool)
        n237 = Not(x=w326) -> (.not. x?=w325:bool)
        n238 = local write "Auto"(w325) -> ()
      }
      event "Auto Start Temp": Value Change {
        n239 = event-data() -> ()  [unwired: 1 in, 6 out]
        n240 = local read "Auto Start Test"() -> (w332:bool)
        n241 = case shown="False" w332 {
          frame False {
            n242 = stacked-sequence {
              frame #0 {
                n243 = local write "START TEMP"(FALSE ("START TEMP")) -> ()
              }
              frame #1 {
                n244 = Wait (ms)(milliseconds to wait=u32 2000) -> ()  [unwired: 1 out]
              }
              frame #2 {
                n245 = local write "Command"("VC;0") -> ()
              }
              frame #3 {
                n246 = Wait (ms)(milliseconds to wait=u32 2000) -> ()  [unwired: 1 out]
              }
              frame #4 {
                w342 = T19."Enabled" ("Disabled")
                (unwired) T24."Imaging" ("Main Dashboard Buttons")
                w343 = "" ("FILE")
                n247 = local write "Main Tab"(T2."Adv Scar" ("Main Tab")) -> ()
                n248 = local write "measured_stroke"(0.0 ("measured_stroke")) -> ()
                n249 = local write "Main Dashboard Buttons"(T1."Imaging" ("Main Dashboard Buttons")) -> ()
                n250 = property on="RUN" class="Bool (strict)"("Visible"=TRUE) -> ()  [unwired: 2 in, 2 out]
                n251 = local write "Command"("VC;0") -> ()
                n252 = local write "TEST FILE NAM,E SAVED"(FALSE ("TEST FILE NAM,E SAVED")) -> ()
                n253 = local write "Fuel Discription :"(w343) -> ()
                n254 = local write "Batch Ref Num :"(w343) -> ()
                n255 = local write "Remarks :"(w343) -> ()
                n256 = local write "FILE"(w343) -> ()
                n257 = property on="FRICVALZ 2" class="Bool (strict)"("DisabledEnum"=w342) -> ()  [unwired: 2 in, 2 out]
                n258 = property on="FRICVALZ 4" class="Bool (strict)"("DisabledEnum"=w342) -> ()  [unwired: 2 in, 2 out]
                n259 = property on="FRICVALZ 3" class="Bool (strict)"("DisabledEnum"=w342) -> ()  [unwired: 2 in, 2 out]
              }
            }
          }
          frame True {
            n260 = flat-sequence {
              frame #0 {
                n261 = local write "Command"("VC;1") -> ()
              }
              frame #1 {
                n262 = Wait (ms)(milliseconds to wait=u32 2000) -> ()  [unwired: 1 out]
              }
              frame #2 {
                n263 = local write "Command"("VC;1") -> ()
              }
              frame #3 {
                n264 = Wait (ms)(milliseconds to wait=u32 2000) -> ()  [unwired: 1 out]
              }
              frame #4 {
                w350 = T19."Disabled" ("Disabled")
                n265 = property on="RUN" class="Bool (strict)"("Visible"=FALSE) -> ()  [unwired: 2 in, 2 out]
                n266 = property on="FRICVALZ 2" class="Bool (strict)"("DisabledEnum"=w350) -> ()  [unwired: 2 in, 2 out]
                n267 = property on="FRICVALZ 4" class="Bool (strict)"("DisabledEnum"=w350) -> ()  [unwired: 2 in, 2 out]
                n268 = property on="FRICVALZ 3" class="Bool (strict)"("DisabledEnum"=w350) -> ()  [unwired: 2 in, 2 out]
                "START TEMP" <- TRUE
              }
            }
          }
        }
      }
      event "FILE", "USERNAME", "USER ID": Mouse Enter {
        n269 = event-data() -> ()  [unwired: 1 in, 4 out]
        n270 = dll-call lib="kernel32.dll" fn="Wow64DisableWow64FsRedirection"("OldValue"=0) -> (error out=w357:errorcluster, "OldValue"=w355:i32)  [unwired: 4 in, 1 out]
        n271 = call <vilib>:"System Exec.vi"("run minimized? (F)"=TRUE, "error in (no error)"=w357, "command line"="C:\\Program Files\\Common Files\\Microsoft Shared\\Ink\\TabTip.exe") -> ("error out"=w356:errorcluster)  [unwired: 5 in, 3 out]
        n272 = dll-call lib="kernel32.dll" fn="Wow64EnableWow64FsRedirection"(error in=w356, "OldValue"=w355) -> ()  [unwired: 4 in, 2 out]
      }
      event "EDIT": Value Change {
        n273 = event-data() -> ()  [unwired: 1 in, 6 out]
        n274 = local read "EDIT"() -> (w358:bool)
        n275 = case shown="False" w358 {
          frame False {
            n276 = control-ref of="This VI"() -> (w375:refnum<vi>)
            n277 = property class="VI"(reference=w375) -> (reference out=w366:refnum<vi>, error out=w370:errorcluster, "Panel"=w374:refnum<vi>)  [unwired: 1 in]
            n278 = property class="Pnl"(reference=w374, error in=w370) -> (reference out=w368:refnum<vi>, error out=w371:errorcluster, "Panes[]"=w373:refnum<vi>[])
            n279 = for {
              tunnel: w373 -> [w381] mode=indexing
              tunnel: T21."Always Off" ("Horizontal Scrollbar Visibility") -> [w380]
              tunnel: w371 -> [w377]
              tunnel: [w376] -> w369
              n280 = property class="Pane"(reference=w381, error in=w377, "HorizScrollbarVisibility"=w380) -> (reference out=w378:refnum<vi>, error out=w379:errorcluster)
              n281 = Close Reference(reference=w378, error in (no error)=w379) -> (error out=w376:errorcluster)
            }
            n282 = Close Reference(reference=w368, error in (no error)=w369) -> (error out=w367:errorcluster)
            n283 = Close Reference(reference=w366, error in (no error)=w367) -> (error out=w361:errorcluster)
            "error out 7" <- w361
            n284 = call <vilib>:"Clear Errors.vi"("error in (no error)"=w361) -> ("error out"=w360:errorcluster)  [unwired: 5 in, 1 out]
            n285 = local write "Service Password enable"(FALSE ("Service Password enable")) -> ()
            n286 = call <userlib>:"Fit VI window to Largest Dec.vi"("error in (no error)"=w360, "border spacing (2 px)"=1) -> ("error out"=w365:errorcluster, "dup VI Ref"=w363:refnum<vi>)  [unwired: 4 in]
            n287 = invoke on="Invoke Node" class="VI" method="FP.Run-Time Position.Maximized"(reference=w363, error in=w365) -> (error out=w364:errorcluster)  [unwired: 2 in, 3 out]
            n288 = call <vilib>:"Clear Errors.vi"("error in (no error)"=w364) -> ()  [unwired: 5 in, 2 out]
          }
          frame True {
          }
        }
      }
      event "Heater Button": Value Change {
        n289 = event-data() -> ()  [unwired: 1 in, 6 out]
        n290 = local read "Heater Button"() -> (w382:bool)
        n291 = case shown="True" w382 {
          frame True {
            n292 = stacked-sequence {
              frame #0 {
                n293 = Wait (ms)(milliseconds to wait=u32 1500) -> ()  [unwired: 1 out]
              }
              frame #1 {
                n294 = local read "Set Temp"() -> (w384:dbl)
                n295 = Number To Fractional String(number=w384, precision (6)=i16 2) -> (F-format string=w387:string)  [unwired: 2 in]
                n296 = Concatenate Strings("ST;" ("Command"), w387) -> (w386:string)
                n297 = local write "Command"(w386) -> ()
              }
              frame #2 {
                n298 = Wait (ms)(milliseconds to wait=u32 1500) -> ()  [unwired: 1 out]
              }
              frame #3 {
                n299 = local write "Command"("HE;1" ("Command")) -> ()
              }
              frame #4 {
                n300 = Wait (ms)(milliseconds to wait=u32 1500) -> ()  [unwired: 1 out]
              }
              frame #5 {
                n301 = stacked-sequence {
                  frame #0 {
                    n302 = Wait (ms)(milliseconds to wait=u32 1500) -> ()  [unwired: 1 out]
                  }
                  frame #1 {
                    n303 = local read "Set Temp"() -> (w393:dbl)
                    n304 = Number To Fractional String(number=w393, precision (6)=i16 2) -> (F-format string=w396:string)  [unwired: 2 in]
                    n305 = Concatenate Strings("ST;" ("Command"), w396) -> (w395:string)
                    n306 = local write "Command"(w395) -> ()
                  }
                  frame #2 {
                    n307 = Wait (ms)(milliseconds to wait=u32 1500) -> ()  [unwired: 1 out]
                  }
                  frame #3 {
                    n308 = local write "Command"("HE;1" ("Command")) -> ()
                  }
                  frame #4 {
                    n309 = Wait (ms)(milliseconds to wait=u32 1500) -> ()  [unwired: 1 out]
                  }
                }
              }
            }
          }
          frame False {
            n310 = stacked-sequence {
              frame #0 {
                n311 = Wait (ms)(milliseconds to wait=u32 1500) -> ()  [unwired: 1 out]
              }
              frame #1 {
                n312 = Concatenate Strings("ST;" ("Command"), "0" ("string")) -> (w403:string)
                n313 = local write "Command"(w403) -> ()
              }
              frame #2 {
                n314 = Wait (ms)(milliseconds to wait=u32 1500) -> ()  [unwired: 1 out]
              }
              frame #3 {
                n315 = local write "Command"("HE;0" ("Command")) -> ()
              }
              frame #4 {
                n316 = Wait (ms)(milliseconds to wait=u32 1500) -> ()  [unwired: 1 out]
              }
            }
          }
        }
      }
      event "Headen Service Button": Value Change {
        n317 = event-data() -> ()  [unwired: 1 in, 6 out]
        n318 = local read "Headen Service Button"() -> (w408:bool)
        n319 = case shown="True" w408 {
          frame False {
            n320 = property on="Password 3" class="Clust (strict)"("Visible"=FALSE) -> ()  [unwired: 2 in, 2 out]
            n321 = property on="Service Password Log" class="Str"("Visible"=FALSE) -> ()  [unwired: 2 in, 2 out]
          }
          frame True {
            n322 = property on="Password 3" class="Clust (strict)"("Visible"=TRUE) -> ()  [unwired: 2 in, 2 out]
            n323 = property on="Service Password Log" class="Str"("Visible"=TRUE) -> ()  [unwired: 2 in, 2 out]
          }
        }
      }
      event "Password 3.Service Password": Value Change {
        n324 = event-data() -> ()  [unwired: 1 in, 6 out]
